vi "Setup.vi"(0 "RFSG Cable Path in":refnum<class "SG Abstract Path.lvclass">, 11 "error in (no error)":errorcluster) -> (4 "RFSG Cable Path out":refnum<class "SG Abstract Path.lvclass">, 15 "error out":errorcluster)   [LabVIEW 2023, in "RFFixtureCharact.Public.lvlib" / "SG Abstract Path.lvclass"]
uses:
  SG Abstract Path.lvclass
  C:/srd-semi-rfcal-software/AuxTools/STSRFFixtureCharactUtility/Source/Code Modules/Common/Base Classes/Path/Path.lvclass
  Instruments/Power Meter/Power Meter Base/Power Meter Base.lvclass
  Scalar Path/Scalar Path.lvclass
  Instruments/Power Meter/Power Meter Factory/Power Meter Factory.lvclass
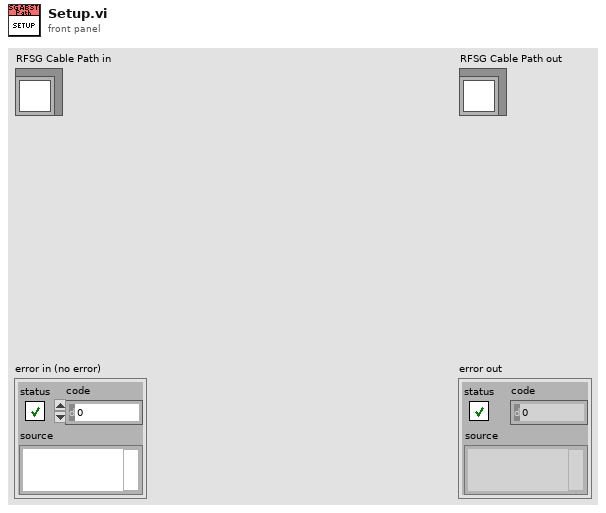
[diagram p1: front panel]
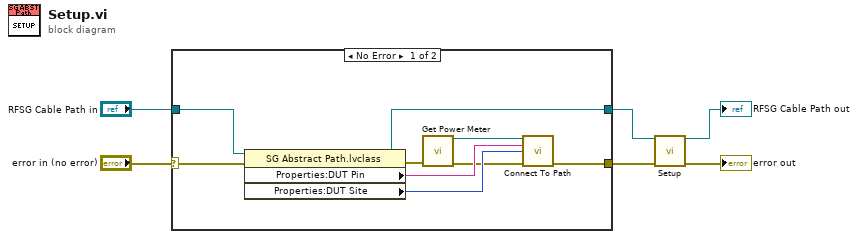
[diagram p0: block diagram]
diagram:
  n1 = case shown="No Error" "error in (no error)" {
    selector: "error in (no error)" -> [w7 w17]
    tunnel: "RFSG Cable Path in" -> [w13 w16]
    tunnel: [w12 w16] -> w4
    tunnel: [w15 w17] -> w3
    frame No Error {
      n2 = property class="SG Abstract Path.lvclass"(reference=w13, error in=w7) -> (reference out=w12:refnum<class "SG Abstract Path.lvclass">, error out=w9:errorcluster, "Properties:DUT Pin"=w11:string, "Properties:DUT Site"=w10:i32)
      n3 = call "Get Power Meter.vi"("error in (no error)"=w9) -> ("Power Meter Base out"=w14:refnum<class "Power Meter Base.lvclass">, "error out"=w8:errorcluster)  [unwired: 13 in]
      n4 = call-dynamic "Connect To Path.vi"("Power Meter Base in"=w14, "DUT Pin"=w11, "DUT Site"=w10, "error in"=w8) -> ("error out"=w15:errorcluster)  [unwired: 10 in, 1 out]
    }
    frame Error {
    }
  }
  n5 = call-parent "Setup.vi"("Scalar Path in"=w4, "error in (no error)"=w3) -> ("Scalar Path out"=→"RFSG Cable Path out":refnum<class "SG Abstract Path.lvclass">, "error out"=→"error out":errorcluster)  [unwired: 12 in]
